vi "_handshake.vi"(8 "error in (no error)":errorcluster, 11 "rethinkdb in":refnum<class "rethinkdb.lvclass">) -> (0 "error out":errorcluster, 3 "rethinkdb out":refnum<class "rethinkdb.lvclass">)   [LabVIEW 2017, in "rethinkdb.lvclass"]
uses:
  rethinkdb.lvclass
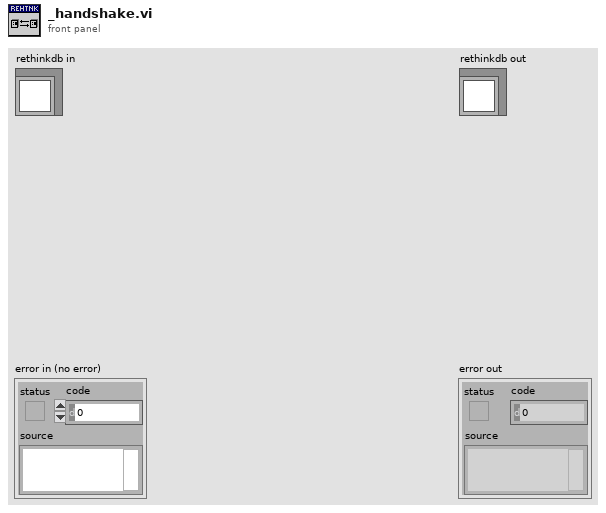
[diagram p1: front panel]
types:
  T1 = typedef "rethinkdb_settings.ctl" = cluster{"host":string, "port":u16, "user":string, "password":string, "timeout":i32, "db":string}
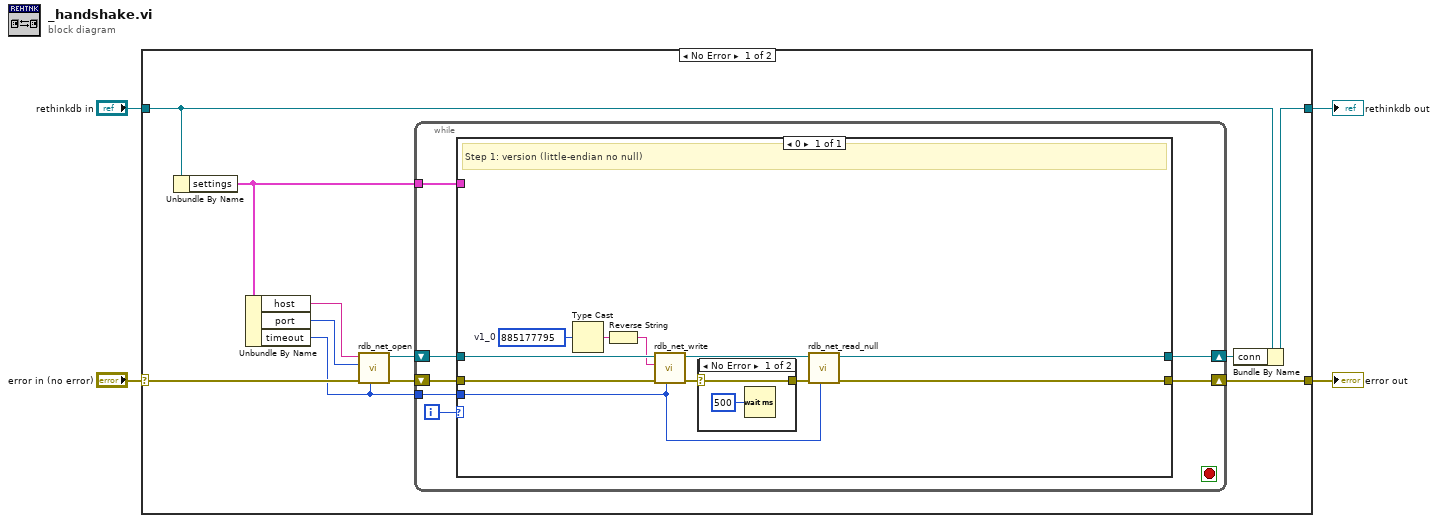
[diagram p0: block diagram]
diagram:
  n1 = case shown="No Error" "error in (no error)" {
    selector: "error in (no error)" -> [w14 w38]
    tunnel: [w9 w38] -> w3
    tunnel: [w11 w37] -> w1
    tunnel: "rethinkdb in" -> [w15 w37]
    frame No Error {
      n2 = Unbundle By Name(w15) -> ("settings"=w6:T1)
      n3 = Unbundle By Name(w6) -> ("host"=w13:string, "port"=w12:u16, "timeout"=w7:i32)
      n4 = call "rdb_net_open.vi"("timeout ms (10000)"=w7, "error in (no error)"=w14, "port (28015)"=w12, "host (\"localhost\")"=w13) -> ("error out"=w10:errorcluster, "conn out"=w8:refnum<k5>)  [unwired: 6 in]
      n5 = while {
        tunnel: w7 -> [w19]
        shift-right: [w21] -> w9
        shift-left: w10 -> [w22]
        shift-right: [w17] -> w5
        shift-left: w8 -> [w20]
        tunnel: w6 -> [w16]
        i -> [w18]
        stop <- _ stop-if-true
        n6 = case shown="0" w18 {
          tunnel: w22 -> [w30]
          tunnel: [w29] -> w21
          tunnel: w20 -> [w28]
          tunnel: w19 -> [w25]
          tunnel: [w23] -> w17
          tunnel: w16 -> [_]
          frame 0 {
            w27 = 885177795  # v1_0
            # "Step 1: version (little-endian no null)"
            n7 = Type Cast(x=w27) -> (*(type *) &x=w26:string)  [unwired: 1 in]
            n8 = Reverse String(1:w26) -> (0:w24:string)
            n9 = call "rdb_net_write.vi"("timeout ms (10000)"=w25, "error in (no error)"=w30, "data in"=w24, "conn in"=w28) -> ("error out"=w31:errorcluster, "conn out"=w33:refnum<k5>)  [unwired: 5 in, 1 out]
            n10 = case shown="No Error" w31 {
              selector: w31 -> [w34 w36]
              tunnel: [w34 w36] -> w32
              frame No Error {
                n11 = Wait (ms)(milliseconds to wait=u32 500) -> ()  [unwired: 1 out]
              }
              frame Error {
              }
            }
            n12 = call "rdb_net_read_null.vi"("timeout ms (10000)"=w25, "error in (no error)"=w32, "conn in"=w33) -> ("error out"=w29:errorcluster, "conn out"=w23:refnum<k5>)  [unwired: 6 in, 1 out]
          }
        }
      }
      n13 = Bundle By Name(cluster=w15, "conn"=w5) -> (w11:refnum<class "rethinkdb.lvclass">)
    }
    frame Error {
    }
  }
  "error out" <- w3
  "rethinkdb out" <- w1
